vi "GoToNearBallPlacementSkill.vi"(8 "error in (no error)":errorcluster, 9 "Game":refnum<class "Game.lvclass">, 10 "Robot":refnum<class "Robot.lvclass">, 11 "GoToNearBallPlacementSkill in":refnum<class "GoToNearBallPlacementSkill.lvclass">) -> (0 "error out":errorcluster, 1 "arrive":bool, 2 "Robot out":refnum<class "Robot.lvclass">, 3 "GoToNearBallPlacementSkill out":refnum<class "GoToNearBallPlacementSkill.lvclass">)   [LabVIEW 2020, in "GoToNearBallPlacementSkill.lvclass"]
uses:
  GoToNearBallPlacementSkill.lvclass
  Game_class/Game.lvclass
  Robot_class/Robot.lvclass
  C:/RoboIME/SSL_AI/Object_class/Object.lvclass
  Game_class/Game.lvclass/Game.ctl
  Object_class/Object.lvclass/Object.ctl
  Robot_class/Robot.lvclass/Robot.ctl
  <vilib>/Analysis/coordinate.llb/Wrap Angle (scalar).vi
  Robot_class/Read orientation.vi
  Object_class/Read position(x,y).vi
  Game_class/Read FieldRef.vi
  Game_class/Read BallRef.vi
  Object_class/Read x.vi
  Object_class/Read y.vi
  Game_class/Read Utilities.lvclass.vi
  Robot_class/Write dest_x.vi
  Robot_class/Write dest_y.vi
  Robot_class/Write dest_orientation.vi
  Ball_class/Ball.lvclass
  Utilities_class/Utilities.lvclass
  Field_class/Field.lvclass
  <vilib>/Analysis/NI_AAL_Angle.lvlib
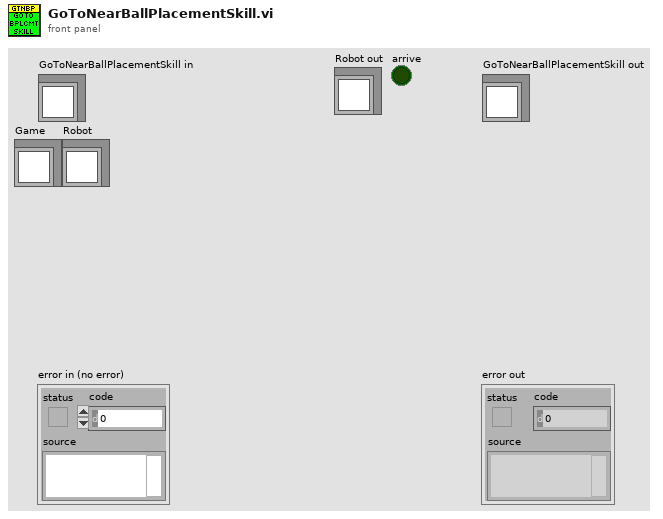
[diagram p1: front panel]
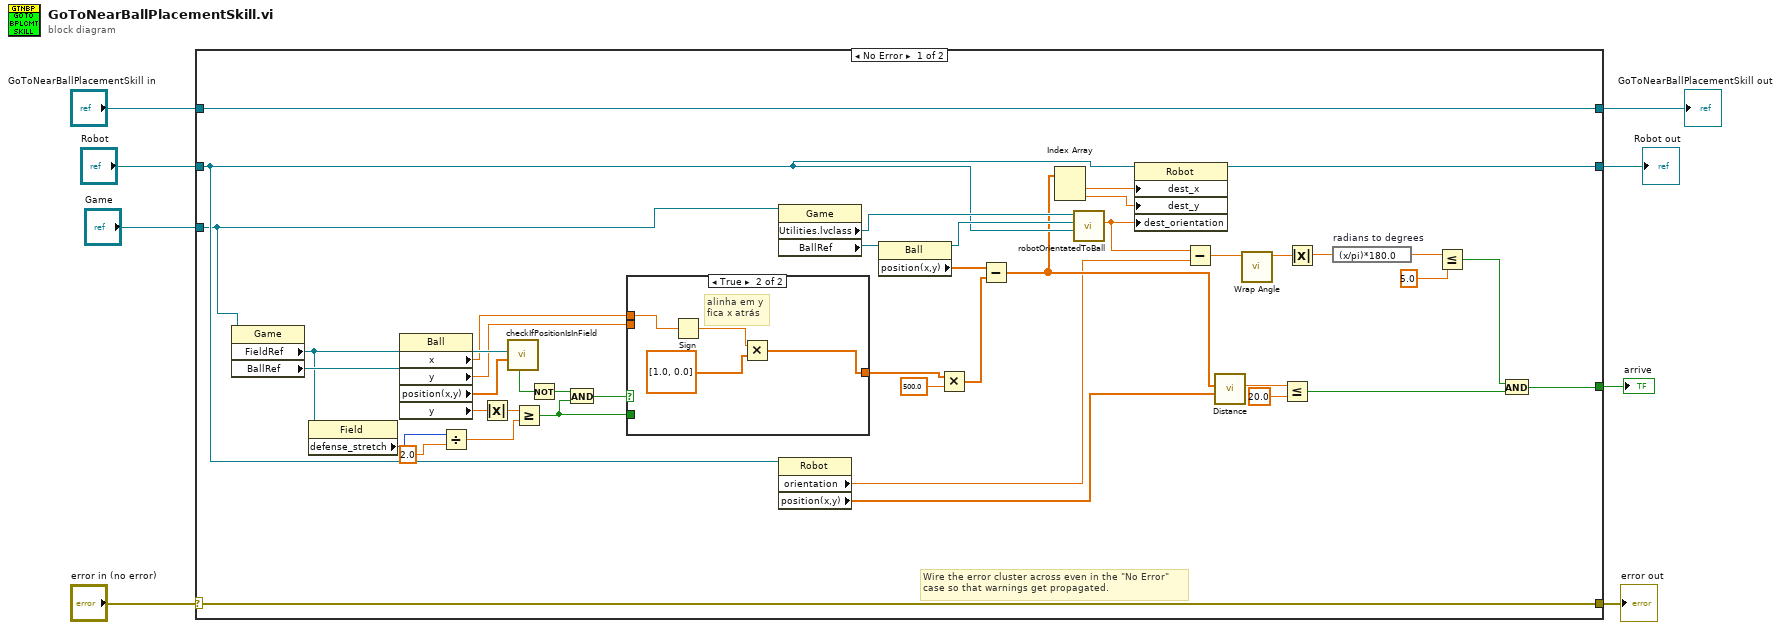
[diagram p0: block diagram]
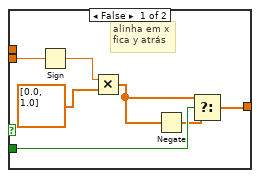
[diagram p2: hidden frame]
diagram:
  n1 = case shown="No Error" "error in (no error)" {
    selector: "error in (no error)" -> [w49 w63]
    tunnel: [w49 w63] -> w7
    tunnel: [w50 w62] -> w5
    tunnel: "GoToNearBallPlacementSkill in" -> [w50 w62]
    tunnel: "Game" -> [w23 _]
    tunnel: "Robot" -> [w39 _]
    tunnel: [w40 _] -> w2
    tunnel: [w25 _] -> w1
    frame No Error {
      # "Wire the error cluster across even in the \"No Error\"\ncase so that warnings get propagated."
      n2 = property class="Game"(reference=w23) -> ("FieldRef"=w16:refnum<class "Field.lvclass">, "BallRef"=w22:refnum<class "Ball.lvclass">)  [unwired: 1 in, 2 out]
      n3 = property class="Field"(reference=w16) -> ("defense_stretch"=w15:i32)  [unwired: 1 in, 2 out]
      n4 = property class="Ball"(reference=w22) -> ("x"=w9:dbl, "y"=w10:dbl, "position(x,y)"=w21:dbl[], "y"=w18:dbl)  [unwired: 1 in, 2 out]
      n5 = Divide(x=w15, y=2.0) -> (x/y=w13:dbl)
      n6 = Absolute Value(x=w18) -> (abs(x)=w17:dbl)
      n7 = call "checkIfPositionIsInField.vi"("Position"=w21, "FieldRef"=w16) -> ("x Is in Field?"=w20:bool)  [unwired: 5 in, 4 out]
      n8 = Greater Or Equal?(x=w17, y=w13) -> (x >= y?=w11:bool)
      n9 = Not(x=w20) -> (.not. x?=w19:bool)
      n10 = And(x=w19, y=w11) -> (x .and. y?=w12:bool)
      n11 = case shown="True" w12 {
        tunnel: [w55 w58] -> w24
        tunnel: w11 -> [w57 _]
        tunnel: w10 -> [w52 _]
        tunnel: w9 -> [_ w60]
        frame False {
          # "alinha em x\nfica y atrás"
          n12 = Sign(1:w52) -> (0:w51:dbl)
          n13 = Multiply(x=w51, y=dbl[] [0.0, 1.0]) -> (x*y=w53:dbl[])
          n14 = Negate(x=w53) -> (-x=w56:dbl[])
          n15 = Select(t=w53, s=w57, f=w56) -> (s? t:f=w55:dbl[])
        }
        frame True {
          # "alinha em y\nfica x atrás"
          n16 = Sign(1:w60) -> (0:w59:dbl)
          n17 = Multiply(x=w59, y=dbl[] [1.0, 0.0]) -> (x*y=w58:dbl[])
        }
      }
      n18 = property class="Game"(reference=w23) -> ("Utilities.lvclass"=w41:refnum<class "Utilities.lvclass">, "BallRef"=w48:refnum<class "Ball.lvclass">)  [unwired: 1 in, 2 out]
      n19 = property class="Robot"(reference=w39) -> ("orientation"=w32:dbl, "position(x,y)"=w38:dbl[])  [unwired: 1 in, 2 out]
      n20 = property class="Ball"(reference=w48) -> (reference out=w42:refnum<class "Ball.lvclass">, "position(x,y)"=w47:dbl[])  [unwired: 1 in, 1 out]
      n21 = Multiply(x=w24, y=500.0) -> (x*y=w45:dbl[])
      n22 = Subtract(x=w47, y=w45) -> (x-y=w37:dbl[])
      n23 = Index Array(array=w37) -> (element #1=w44:dbl, element #2=w43:dbl)  [unwired: 2 in]
      n24 = call "robotOrientatedToBall.vi"("Robot"=w39, "BallRef"=w42, "Utilities in"=w41) -> ("Orientation"=w33:dbl)  [unwired: 6 in, 2 out]
      n25 = property class="Robot"(reference=w39, "dest_x"=w44, "dest_y"=w43, "dest_orientation"=w33) -> (reference out=w40:refnum<class "Robot.lvclass">)  [unwired: 1 in, 1 out]
      n26 = Subtract(x=w33, y=w32) -> (x-y=w31:dbl)
      n27 = call "Distance.vi"("P1"=w38, "P2"=w37) -> ("Distance"=w36:dbl)  [unwired: 7 in, 2 out]
      n28 = call-poly <vilib>:"Wrap Angle.vi"("angle in"=w31) -> ("angle out"=w30:dbl)  [unwired: 9 in, 1 out]
      n29 = Less Or Equal?(x=w36, y=20.0) -> (x <= y?=w34:bool)
      n30 = Absolute Value(x=w30) -> (abs(x)=w29:dbl)
      n31 = expression code="(x/pi)*180.0" "radians to degrees"(w29) -> (w28:dbl)
      n32 = Less Or Equal?(x=w28, y=5.0) -> (x <= y?=w26:bool)
      n33 = And(x=w26, y=w34) -> (x .and. y?=w25:bool)
    }
    frame Error {
    }
  }
  "error out" <- w7
  "GoToNearBallPlacementSkill out" <- w5
  "Robot out" <- w2
  "arrive" <- w1
